vi "SVT Octave Spectrum Conversion.vi"   [LabVIEW 2017, in "SoundVib_Octave.lvlib"]
doc: "Converts an octave spectrum between dB/linear, magnitude/magnitude^2, spectrum/spectral density, and dB ref1/dB ref2. \n\nYou can use this VI to convert one octave spectrum or N octave spectra. Wire data to the <B>octave spectrum</B> input to determine the polymorphic instance to use or manually select the instance."
uses:
  <vilib>/addons/Sound and Vibration/svt_Octave/SoundVib_Octave.lvlib
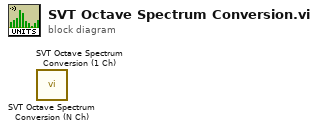
[diagram p0: block diagram]
diagram:
  n1 = call <vilib>:"SVT Octave Spectrum Conversion (N Ch).vi"() -> ()  [unwired: 12 in, 4 out]
  n2 = call <vilib>:"SVT Octave Spectrum Conversion (1 Ch).vi"() -> ()  [unwired: 12 in, 4 out]
